vi "BW.vi"(8 "错误输入（无错误）":errorcluster, 10 "frequency":dbl, 11 "Analog Waveforms":waveform(dbl)[](array[waveform])) -> (0 "错误输出":errorcluster, 3 "Gain Display":cluster{dbl[], dbl[]}(graph)={[2000.0, 4000.0, 6000.0, 8000.0, 10000.0, 12000.0], [0.0, 0.0, 0.0, 0.0, 0.0, 0.0]})   [LabVIEW 2019]
uses:
  <vilib>/Waveform/WDTOps.llb/WDT Index Channel DBL.vi
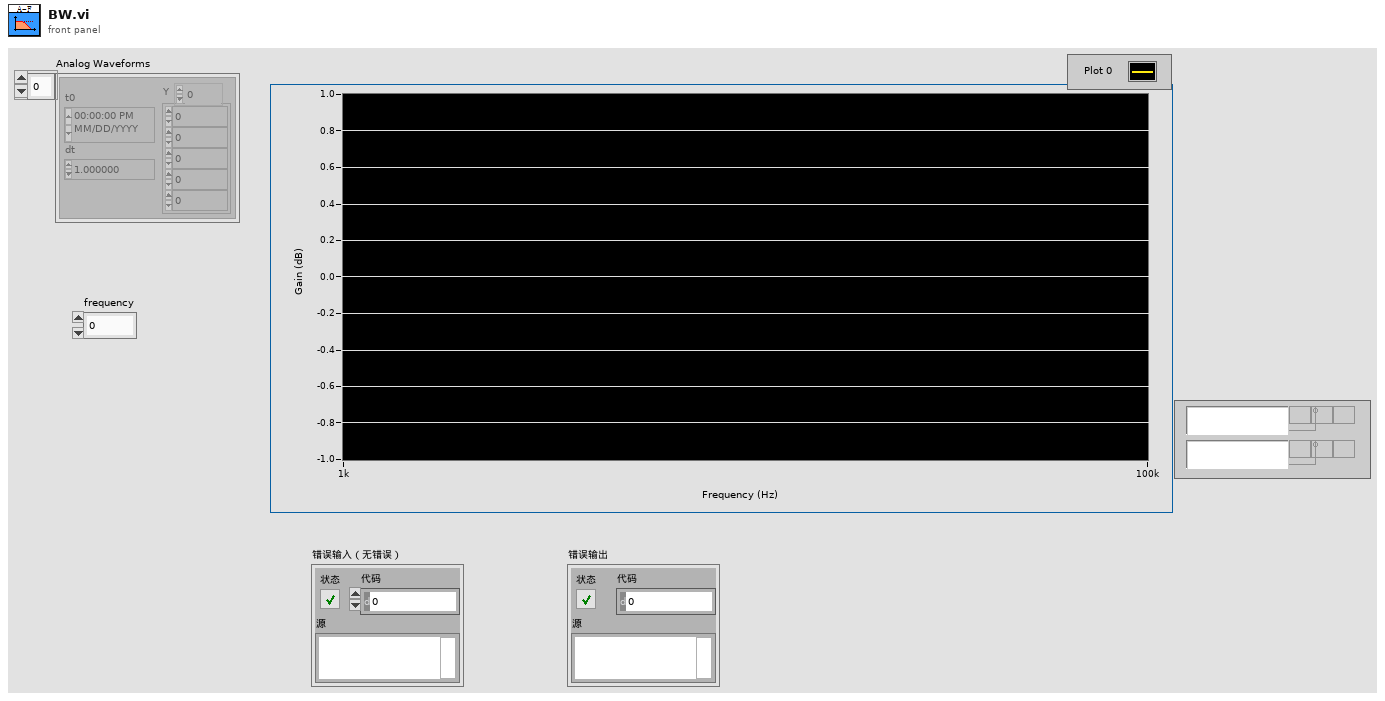
[diagram p1: front panel]
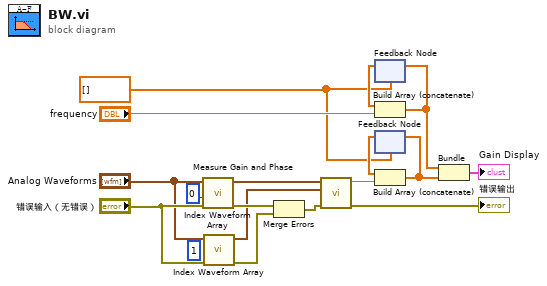
[diagram p0: block diagram]
diagram:
  w1 = dbl[] []
  (unwired) 1 ("index")
  n1 = call-poly <vilib>:"Index Waveform Array.vi"("error in (no error)"="错误输入（无错误）", "index"=0, "waveform array"="Analog Waveforms") -> ("error out"=w16:errorcluster, "waveform"=w12:waveform(dbl))  [unwired: 7 in]
  n2 = call-poly <vilib>:"Index Waveform Array.vi"("error in (no error)"="错误输入（无错误）", "waveform array"="Analog Waveforms") -> ("error out"=w15:errorcluster, "waveform"=w13:waveform(dbl))  [unwired: 8 in]
  n3 = Merge Errors(w16, w15) -> (w17:errorcluster)
  n4 = call "Measure Gain and Phase.vi"("error out输入"=w17, "Ch2"=w13, "Ch1"=w12) -> ("错误输出"=→"错误输出":errorcluster, "Gain (dB)"=w7:dbl)  [unwired: 6 in, 1 out]
  n5 = feedback #1(w1) -> (w3:dbl[])
  n6 = Build Array (concatenate)(w3, "frequency") -> (w9:dbl[])
  n7 = feedback-in #1(w9) -> ()
  n8 = feedback #2(w1) -> (w6:dbl[])
  n9 = Build Array (concatenate)(w6, w7) -> (w8:dbl[])
  n10 = feedback-in #2(w8) -> ()
  n11 = Bundle(w9, w8) -> (→"Gain Display":cluster{dbl[], dbl[]})  [unwired: 1 in]
